vi "Q_Insert.vi"(8 "error in":errorcluster caption="错误输入（无错误）", 10 "Vi Alias":string, 11 "ChildNode*":refnum<data-value>) -> (0 "error out":errorcluster caption="错误输出")   [LabVIEW 2013, in "PanelDataNode.lvclass"]
uses:
  PanelDataNode.lvclass
  PanelDataNode.lvclass/PanelDataNode.ctl
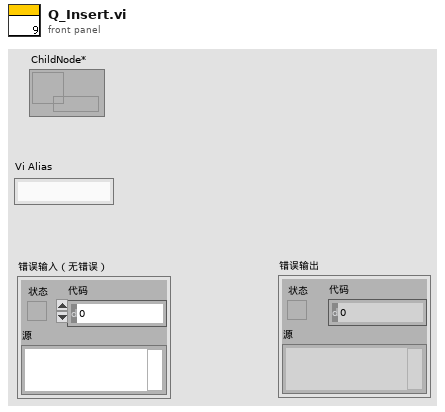
[diagram p1: front panel]
types:
  T1 = cluster{"ChildNode*":refnum<data-value>, "VI*":refnum<vi>}
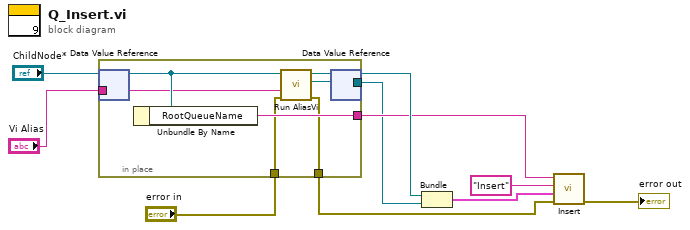
[diagram p0: block diagram]
diagram:
  n1 = in-place {
    in-place-border: [w17] -> w6
    in-place-border: [w14] -> w4
    in-place-border: "Vi Alias" -> [w13]
    in-place-border: [w12] -> w2
    in-place-border: "error in" -> [w11]
    n2 = in-place-dvr #1("ChildNode*") -> (w16:refnum<class "PanelDataNode.lvclass">)  [unwired: 1 out]
    n3 = Unbundle By Name(w16) -> ("RootQueueName"=w17:string)
    n4 = call-dynamic "Run AliasVi.vi"("error in (no error)"=w11, "Vi Alias"=w13, "PanelDataNode 输入"=w16) -> ("error out"=w12:errorcluster, "VI*"=w14:refnum<vi>, "PanelDataNode 输出"=w15:refnum<class "PanelDataNode.lvclass">)  [unwired: 6 in]
    n5 = in-place-dvr #1(w15) -> (w7:refnum<data-value>)  [unwired: 1 out]
  }
  n6 = Bundle("ChildNode*"=w7, "VI*"=w4) -> (w10:T1)  [unwired: 1 in]
  n7 = call "Insert.vi"("error in"=w2, "Data"=w10, "Event"="Insert", "QueueName"=w6) -> ("error out"=→"error out":errorcluster)  [unwired: 6 in, 1 out]
